vi "Read Button.vi"(8 "Error In":errorcluster, 11 "EZ430-Chronos Ref":T2) -> (0 "Error Out":errorcluster, 2 "Buttons":T1, 3 "EZ430-Chronos Config":T2)   [LabVIEW 2011, in "LVH-EZ430.lvlib"]
doc: "Read button data from the EZ430-Chronos. The watch must be transmitting in PPT mode before calling this VI."
uses:
  LVH-EZ430.lvlib
  Private/Type Defs/EZ430-Chronos Ref.ctl
  Private/Type Defs/Buttons.ctl
  Private/Type Defs/Command.ctl
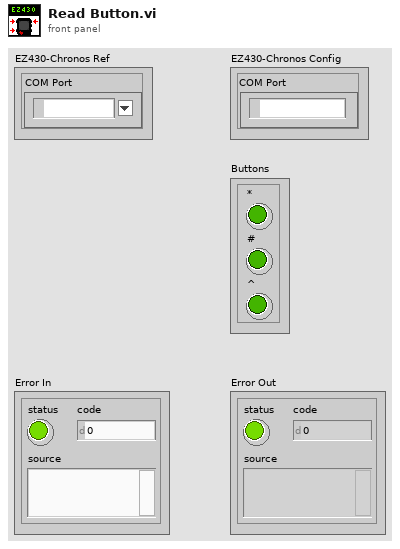
[diagram p1: front panel]
types:
  T1 = typedef "LVH-EZ430.lvlib/Buttons.ctl" = cluster{"*":bool, "#":bool, "^":bool}
  T2 = typedef "LVH-EZ430.lvlib/EZ430-Chronos Ref.ctl" = cluster{"COM Port":refnum<visa-resource-name>}
  T3 = typedef "LVH-EZ430.lvlib/Command.ctl" = enum8{"Get Hardware Status", "Reset RF Access Point", "Start BlueRobin Transmitter", "Set BlueRobin Trans ID", "Get BlueRobin Trans ID", "Set BlueRobin Heart Rate To Transmit", "Stop BlueRobin Transmitter", "Start ACC / PPT Mode", "Read ACC / PPT", "Stop SimpliciTI Stack"}
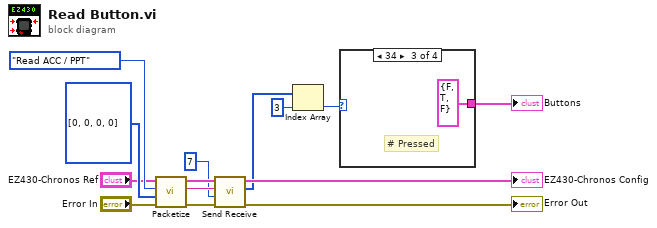
[diagram p0: block diagram]
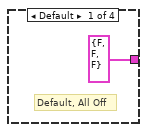
[diagram p2: hidden frame]
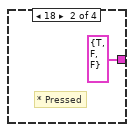
[diagram p3: hidden frame]
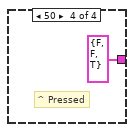
[diagram p4: hidden frame]
diagram:
  n1 = call "Packetize.vi"("Error In"="Error In", "Data"=u8[] [0, 0, 0, 0], "Command"=Command."Read ACC / PPT", "EZ430-Chronos Config"="EZ430-Chronos Ref") -> ("Error Out"=w10:errorcluster, "Packet"=w8:string, "EZ430-Chronos Config"=w9:T2)  [unwired: 5 in]
  n2 = call "Send Receive.vi"("Error In"=w10, "Bytes To Read"=u32 7, "Packet"=w8, "EZ430-Chronos Config"=w9) -> ("Error Out"=→"Error Out":errorcluster, "Data"=w4:u8[], "EZ430-Chronos Config"=→"EZ430-Chronos Config":T2)  [unwired: 5 in]
  n3 = Index Array(array=w4, index=3) -> (element=w2:u8)
  n4 = case shown="34" w2 {
    tunnel: [T1 {"*"=FALSE, "#"=FALSE, "^"=FALSE} ("Buttons") T1 {"*"=TRUE, "#"=FALSE, "^"=FALSE} ("Buttons") T1 {"*"=FALSE, "#"=TRUE, "^"=FALSE} ("Buttons") T1 {"*"=FALSE, "#"=FALSE, "^"=TRUE} ("Buttons")] -> w1
    frame Default {
      # "Default, All Off"
    }
    frame 18 {
      # "* Pressed"
    }
    frame 34 {
      # "# Pressed"
    }
    frame 50 {
      # "^ Pressed"
    }
  }
  "Buttons" <- w1
